vi "enqueue_command.vi"(8 "error in (no error)":errorcluster caption="错误输入（无错误）", 10 "command":cluster{"cmd":T1, "cmd data":variant}, 11 "OneMotion输入":refnum<class "OneMotion.lvclass">) -> (0 "error out":errorcluster caption="错误输出", 3 "OneMotion输出":refnum<class "OneMotion.lvclass">)   [LabVIEW 2016, in "MotionControl.lvlib" / "OneMotion.lvclass"]
uses:
  <userlib>/MotionControl/OneMotion/OneMotion.lvclass
  <userlib>/MotionControl/OneMotion/cmd_motion.ctl
  <userlib>/MotionControl/OneMotion/OneMotion.lvclass/OneMotion.ctl
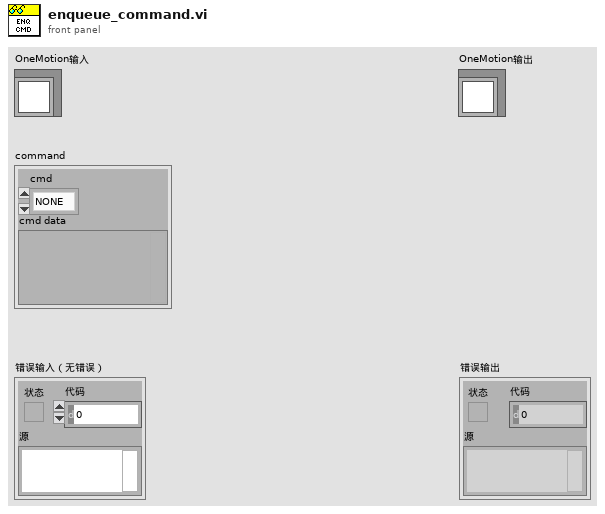
[diagram p1: front panel]
types:
  T1 = typedef "MotionControl.lvlib/OneMotion.lvclass/cmd_motion.ctl" = enum16{"NONE", "MOVE_MOTION", "EXIT", "STP_MOTION", "SPEED_MOTION", "WAIT_FOR_S3", "WAIT_A_TIME", "SKIP"}
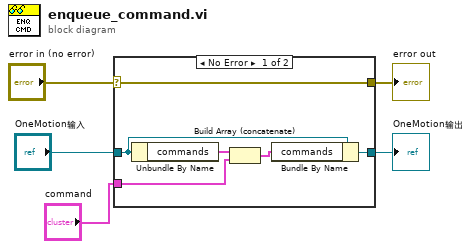
[diagram p0: block diagram]
diagram:
  n1 = case shown="No Error" "error in (no error)" {
    selector: "error in (no error)" -> [w11 w12]
    tunnel: [w11 w12] -> w4
    tunnel: [w9 w13] -> w2
    tunnel: "OneMotion输入" -> [w10 w13]
    tunnel: "command" -> [w7 _]
    frame No Error {
      n2 = Unbundle By Name(w10) -> ("commands"=w8:cluster{"cmd":T1, "cmd data":variant}[])
      n3 = Build Array (concatenate)(w8, w7) -> (w6:cluster{"cmd":T1, "cmd data":variant}[])
      n4 = Bundle By Name(cluster=w10, "commands"=w6) -> (w9:refnum<class "OneMotion.lvclass">)
    }
    frame Error {
    }
  }
  "error out" <- w4
  "OneMotion输出" <- w2
